vi "refRidders Zero Finder.vi"(5 "Variant":variant, 6 "accuracy":dbl=1e-08, 7 "level":dbl, 9 "end":dbl=1.0, 10 "start":dbl, 11 "function refnum":T1) -> (0 "error":i32, 2 "f(zero)":dbl, 3 "zero":dbl)   [LabVIEW 2020, in "NI_Gmath.lvlib"]
doc: "Determines a zero of a 1D function in a given interval. The function has to be continuous and has to have different signs at the end points of the interval."
uses:
  NI_Gmath.lvlib
  functionRefnum.ctl
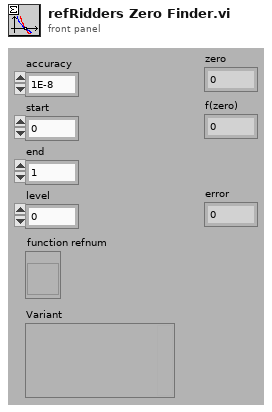
[diagram p1: front panel]
types:
  T1 = typedef "NI_Gmath.lvlib/functionRefnum.ctl" = refnum<vi>
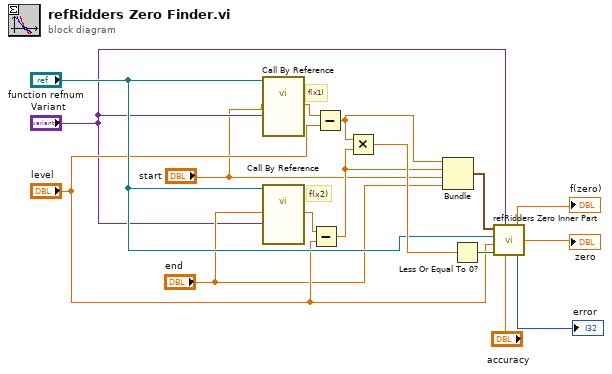
[diagram p0: block diagram]
diagram:
  # "f(x1)"
  # "f(x2)"
  n1 = call-by-ref "?"(reference="function refnum", "Variant"="Variant", "x"="start") -> ("f(x)"=w1:dbl)  [unwired: 4 in, 2 out]
  n2 = call-by-ref "?"(reference="function refnum", "Variant"="Variant", "x"="end") -> ("f(x)"=w5:dbl)  [unwired: 4 in, 2 out]
  n3 = Subtract(x=w5, y="level") -> (x-y=w7:dbl)
  n4 = Subtract(x=w1, y="level") -> (x-y=w8:dbl)
  n5 = Multiply(x=w8, y=w7) -> (x*y=w13:dbl)
  n6 = Bundle(w8, w7, "start"="start", "end"="end") -> (w10:cluster{dbl, dbl, "start":dbl, "end":dbl})  [unwired: 1 in]
  n7 = Less Or Equal To 0?(x=w13) -> (x <= 0?=w12:bool)
  n8 = call "refRidders Zero Inner Part.vi"("start/end/f(x)"=w10, "Variant"="Variant", "function refnum"="function refnum", "level"="level", "accuracy"="accuracy", "case"=w12) -> ("y value"=→"f(zero)":dbl, "end"=→"zero":dbl, "error"=→"error":i32)
